vi "Stop Command.vi"(8 "error in (no error)":errorcluster, 11 "Command Processor in":refnum<class "Command Processor.lvclass">) -> (0 "error out":errorcluster, 3 "Command Processor out":refnum<class "Command Processor.lvclass">)   [LabVIEW 2013, in "Command Processor.lvlib" / "Command Processor.lvclass"]
uses:
  Command Processor.lvclass
  Command Processor.lvclass/Command Processor.ctl
  <vilib>/ActorFramework/Message Enqueuer/Message Enqueuer.lvclass/Message Enqueuer.ctl
  <vilib>/ActorFramework/Message Enqueuer/Enqueue.vi
  <vilib>/ActorFramework/Message Priority Queue/Priority Enqueue.vi
  <vilib>/ActorFramework/Stop Msg/Stop Msg.lvclass
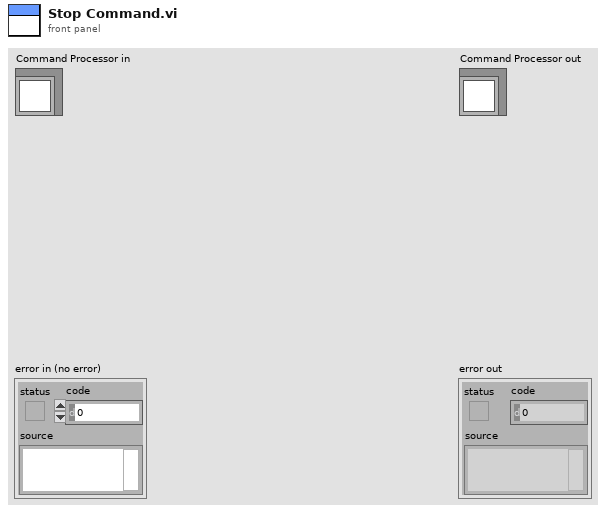
[diagram p1: front panel]
types:
  T1 = typedef "Command Processor.lvlib/Command Processor.lvclass/Command Processor Status.ctl" = cluster{"State Entry time":timestamp, "State Status":T2, "Command Processor Current State":string, "Command Status":T4}
  T2 = typedef "Current Previous State Status.ctl" = cluster{"Current State Status":T3, "Previous State Status":T3}
  T3 = typedef "State Status.ctl" = cluster{"State Name":string, "State Entry Time":timestamp, "State Exit Time":timestamp}
  T4 = typedef "Command Processor.lvlib/Command.lvlib/Command.lvclass/Command Status.ctl" = cluster{"Command Name":string, "Current State Status":T5, "Command Start Time":timestamp, "Command End Time":timestamp, "Previous State Status":T5}
  T5 = typedef "Command Processor.lvlib/Command.lvlib/Command.lvclass/State Status.ctl" = cluster{"State Name":string, "State Entry Time":timestamp, "State Exit Time":timestamp}
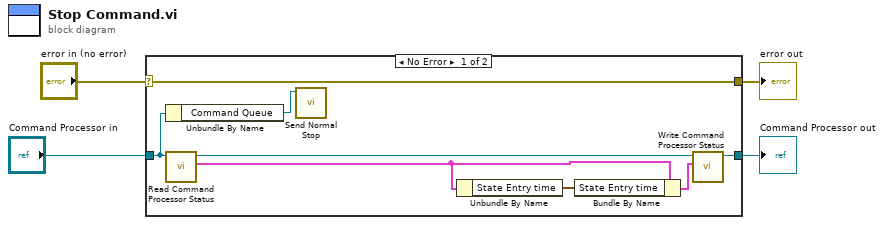
[diagram p0: block diagram]
diagram:
  n1 = case shown="No Error" "error in (no error)" {
    selector: "error in (no error)" -> [w12 w14]
    tunnel: [w12 w14] -> w3
    tunnel: [w8 w13] -> w1
    tunnel: "Command Processor in" -> [w10 w13]
    frame No Error {
      n2 = Unbundle By Name(w10) -> ("Command Queue"=w11:refnum<class "Message Enqueuer.lvclass">)
      n3 = call-dynamic "Read Command Processor Status.vi"("Command Processor in"=w10) -> ("Command Processor Status"=w7:T1, "Command Processor out"=w9:refnum<class "Command Processor.lvclass">)  [unwired: 8 in, 1 out]
      n4 = call <vilib>:"Send Normal Stop.vi"("Message Enqueuer"=w11) -> ()  [unwired: 10 in, 1 out]
      n5 = Unbundle By Name(w7) -> ("State Entry time"=w5:timestamp)
      n6 = Bundle By Name(cluster=w7, "State Entry time"=w5) -> (w6:T1)
      n7 = call-dynamic "Write Command Processor Status.vi"("Command Processor Status"=w6, "Command Processor in"=w9) -> ("Command Processor out"=w8:refnum<class "Command Processor.lvclass">)  [unwired: 8 in, 1 out]
    }
    frame Error {
    }
  }
  "error out" <- w3
  "Command Processor out" <- w1
